vi "UpdateExecutionSettings.vi"(8 "error in (no error)":errorcluster, 11 "Array in":T1[](array[typedef])) -> (0 "error out":errorcluster, 3 "Array out":T1[](array[typedef]))   [LabVIEW 2014, in "control module data interface generator.lvlib"]
uses:
  control module data interface generator.lvlib
  Controls/initialized references.ctl
  Controls/interface VI type.ctl
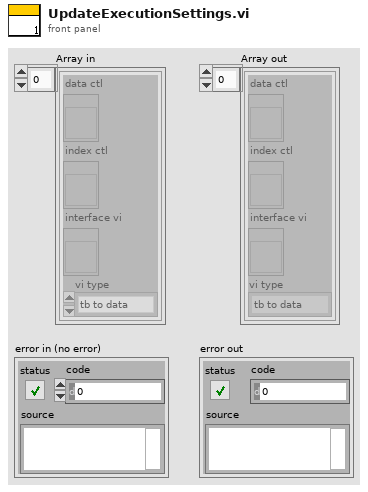
[diagram p1: front panel]
types:
  T1 = typedef "control module data interface generator.lvlib/initialized references.ctl" = cluster{"data ctl":refnum<vi>, "index ctl":refnum<vi>, "interface vi":refnum<vi>, "vi type":T2}
  T2 = typedef "control module data interface generator.lvlib/interface VI type.ctl" = enum16{"tb to data", "data to tb"}
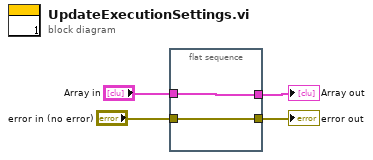
[diagram p0: block diagram]
diagram:
  n1 = flat-sequence {
    tunnel: [w6] -> w1
    tunnel: "Array in" -> [w6]
    tunnel: [w5] -> w3
    tunnel: "error in (no error)" -> [w5]
    frame #0 {
    }
  }
  "error out" <- w3
  "Array out" <- w1
